vi "Handle Heater PIDs.vi"(7 "DataIndex":i32, 8 "Subtag":string="heater", 10 "HeaterTag":string, 11 "gController in":refnum<class "gController.lvclass">) -> ()   [LabVIEW 2017, in "Controller.lvlib" / "gController.lvclass"]
uses:
  gController.lvclass
  C:/Program Files (x86)/National Instruments/LabVIEW 2017/vi.lib/MSR Consulting, LLC/General Reuse/SuperActor/SuperActor.lvclass
  C:/Program Files (x86)/National Instruments/LabVIEW 2017/vi.lib/ActorFramework/Actor/Actor.lvclass
  <vilib>/Platform/TimedLoop/XDataNode/timing_clust.ctl
  <vilib>/Platform/TimedLoop/XDataNode/nitl_modes.ctl
  <vilib>/Platform/TimedLoop/XDataNode/wakeup.ctl
  <vilib>/MSR Consulting, LLC/General Reuse/SuperActor/SuperActor.lvclass/SuperActor.ctl
  gController.lvclass/gController.ctl
  <vilib>/ActorFramework/Actor/Actor.lvclass/Actor.ctl
  <vilib>/ActorFramework/Message Enqueuer/Message Enqueuer.lvclass/Message Enqueuer.ctl
  Messages/Update Heater DC MSG/Update Heater DC MSG.lvclass
  C:/Program Files (x86)/National Instruments/LabVIEW 2017/vi.lib/ActorFramework/Message/Message.lvclass
  Data/SOAP Data.lvclass
  Data/SOAP Data.lvclass/SOAP Data.ctl
  Data/Read temperatures.vi
  <vilib>/MSR Consulting, LLC/General Reuse/SuperActor/Read CVT Session.vi
  Read DataMap.vi
  Read shutdown.vi
  <vilib>/ActorFramework/Message Enqueuer/Init from Existing Queue.vi
  <vilib>/ActorFramework/Message Priority Queue/Priority Enqueue.vi
  <vilib>/addons/control/pid/pid.llb/PID (DBL).vi
  <vilib>/Platform/TimedLoop/XDataNode/XDataNode.xnode
  <vilib>/ActorFramework/Message Enqueuer/Message Enqueuer.lvclass
  <vilib>/MSR Consulting, LLC/General Reuse/Session APIs/_Session Fwk/Session - Root.lvclass
  <vilib>/Platform/TimedLoop/XDataNode/XDNodeRunTimeDep.lvlib
  <vilib>/ActorFramework/Actor/Actor.lvclass
  <vilib>/MSR Consulting, LLC/General Reuse/Session APIs/CVT/CVT.lvclass
  <vilib>/addons/control/pid/NI_PID_pid.lvlib
  <vilib>/ptbypt/NI_PtbyPt.lvlib
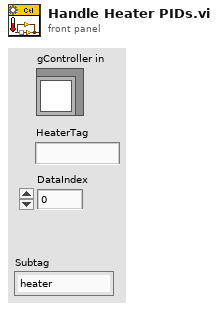
[diagram p1: front panel]
types:
  T1 = typedef "Session - Root.lvclass/Session Handle.ctl" = refnum<data-value>
  T2 = typedef "XDNodeRunTimeDep.lvlib/timing_clust.ctl" = cluster{"Expected End [f-1]":u64, "Actual End [f-1]":u64, "Finished Late? [f-1]":bool, "Expected End [i-1]":u64, "Actual End [i-1]":u64, "Finished Late? [i-1]":bool, "Expected Start [i]":u64, "Actual Start [i]":u64, "Expected Start [f]":u64, "Actual Start [f]":u64, "Source Name":string, "Structure Name":string, "Period":i64, "Deadline":i64, "Offset":i64, "Start":i64, "Priority":i32, "Timeout":i32, "Mode":T3, "Wakeup Reason":T4, "Error":errorcluster, "Source Type":string, "Secondary Source Type":string, "Global End Time":u64, "Global Start Time":u64, "Frame Duration":u64, "Iteration Duration":u64, "Assigned CPU":i32, "I/O Scan Engine Mode":u32}
  T3 = typedef "XDNodeRunTimeDep.lvlib/nitl_modes.ctl" = enum32{"No Change", "Process missed periods, maintain original phase", "Discard missed periods, maintain original phase", "Process missed periods, ignore original phase", "Discard missed periods, ignore original phase"}
  T4 = typedef "XDNodeRunTimeDep.lvlib/wakeup.ctl" = enum32{"Normal", "Aborted", "Asynchronous wakeup", "Timing source error", "Timed loop error", "Timeout"}
  T5 = cluster{"pas_cell_1":sgl, "pas_cell_2":sgl, "pas_las_head_1":sgl, "pas_las_head_2":sgl, "cjc0":sgl, "box_exit":sgl, "crd_heater":sgl, "box_inlet":sgl, "crd_laser_head":sgl, "cjc1":sgl}
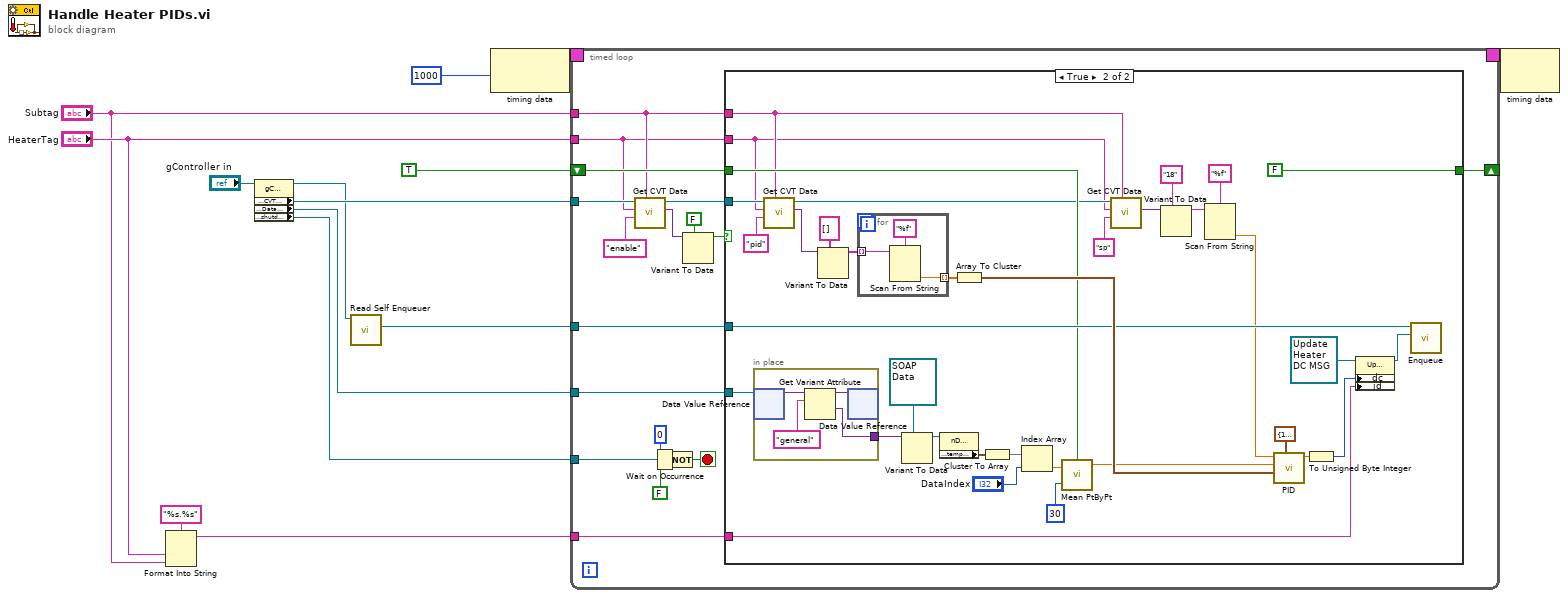
[diagram p0: block diagram]
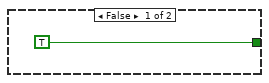
[diagram p2: hidden frame]
diagram:
  n1 = Format Into String(format string="%s.%s", "HeaterTag", "Subtag") -> (resulting string=w6:string)  [unwired: 2 in, 1 out]
  n2 = property class="gController"(reference="gController in") -> (reference out=w3:refnum<class "gController.lvclass">, "Accessors:CVT Session"=w12:T1, "Accessors:DataMap"=w10:refnum<data-value>, "Accessors:shutdown"=w2:refnum<k4>)  [unwired: 1 in, 1 out]
  n3 = call <vilib>:"Read Self Enqueuer.vi"("Actor"=w3) -> ("Self Enqueuer"=w11:refnum<class "Message Enqueuer.lvclass">)  [unwired: 10 in]
  n4 = node-c288(i64 1000 ("Period")) -> (w14:T2)
  n5 = timed-loop {
    timing: w14 -> [_]
    timing-out: [_] -> w13
    tunnel: w12 -> [w17]
    tunnel: "HeaterTag" -> [w15]
    tunnel: w11 -> [w23]
    tunnel: w10 -> [w22]
    tunnel: "Subtag" -> [w16]
    tunnel: w6 -> [w21]
    tunnel: w2 -> [w29]
    shift-right: [w19] -> _
    shift-left: TRUE -> [w20]
    stop <- w28 stop-if-true
    n6 = call <vilib>:"Get CVT Data.vi"("Subgroup"=w16, "Variable"="enable", "Group"=w15, "CVT Session In"=w17) -> ("Data Out"=w26:variant, "CVT Session Out"=w18:T1)  [unwired: 4 in, 2 out]
    n7 = Wait on Occurrence(1:FALSE ("ignore previous (T)"), 2:w29, 3:0 ("ms timeout (-1)")) -> (0:w30:bool)
    n8 = Not(x=w30) -> (.not. x?=w28:bool)
    n9 = Variant To Data(type=FALSE, Variant=w26) -> (data=w27:bool)  [unwired: 1 in, 1 out]
    n10 = case shown="True" w27 {
      tunnel: w23 -> [_ w66]
      tunnel: w22 -> [_ w61]
      tunnel: w21 -> [_ w55]
      tunnel: w20 -> [_ w51]
      tunnel: [TRUE FALSE] -> w19
      tunnel: w18 -> [_ w47]
      tunnel: w16 -> [_ w35]
      tunnel: w15 -> [_ w34]
      frame False {
      }
      frame True {
        n11 = in-place {
          in-place-border: [w72] -> w60
          n12 = in-place-dvr #1(w61) -> (w75:variant)  [unwired: 1 out]
          n13 = Get Variant Attribute(Variant=w75, name="general") -> (duplicate Variant=w74:variant, value=w72:variant)  [unwired: 2 in, 2 out]
          n14 = in-place-dvr #1(w74) -> ()  [unwired: 2 out]
        }
        n15 = call <vilib>:"Get CVT Data.vi"("Subgroup"=w35, "Variable"="pid", "Group"=w34, "CVT Session In"=w47) -> ("Data Out"=w42:variant, "CVT Session Out"=w45:T1)  [unwired: 4 in, 2 out]
        n16 = Variant To Data(type=string[] [], Variant=w42) -> (data=w43:string[])  [unwired: 1 in, 1 out]
        n17 = for {
          tunnel: w43 -> [w71] mode=indexing
          tunnel: [w69] -> w39 mode=indexing
          n18 = Scan From String(format string="%f", input string=w71) -> (output 1=w69:dbl)  [unwired: 3 in, 3 out]
        }
        n19 = Variant To Data(type=refnum<class "SOAP Data.lvclass"> refnum ("Controller.lvlib:nData"), Variant=w60) -> (data=w58:refnum<class "SOAP Data.lvclass">)  [unwired: 1 in, 1 out]
        n20 = property class="nData"(reference=w58) -> ("Accessors:temperatures"=w57:T5)  [unwired: 1 in, 2 out]
        n21 = Array To Cluster(array=w39) -> (cluster=w67:cluster{"[0]":dbl, "[1]":dbl, "[2]":dbl})
        n22 = Cluster To Array(cluster=w57) -> (array=w56:sgl[])
        n23 = Index Array(array=w56, index="DataIndex") -> (element=w53:sgl)
        n24 = call <vilib>:"Mean PtByPt.vi"("x"=w53, "sample length"=30, "initialize"=w51) -> ("mean"=w52:dbl)  [unwired: 1 in, 1 out]
        n25 = call <vilib>:"Get CVT Data.vi"("Subgroup"=w35, "Variable"="sp", "Group"=w34, "CVT Session In"=w45) -> ("Data Out"=w40:variant)  [unwired: 4 in, 3 out]
        n26 = Variant To Data(type="18", Variant=w40) -> (data=w37:string)  [unwired: 1 in, 1 out]
        n27 = Scan From String(format string="%f", input string=w37) -> (output 1=w36:dbl)  [unwired: 3 in, 3 out]
        n28 = call-poly <vilib>:"PID.vi"("output range"=cluster{"output high":dbl, "output low":dbl} {"output high"=100.0, "output low"=0.0}, "PID gains"=w67, "process variable"=w52, "setpoint"=w36) -> ("output"=w64:dbl)  [unwired: 6 in, 1 out]
        n29 = To Unsigned Byte Integer(number=w64) -> (unsigned 8bit integer=w63:u8)
        n30 = property class="Update Heater DC MSG"(reference=refnum<class "Update Heater DC MSG.lvclass"> refnum ("Controller.lvlib:Update Heater DC MSG"), "dc"=w63, "id"=w55) -> (reference out=w62:refnum<class "Update Heater DC MSG.lvclass">)  [unwired: 1 in, 1 out]
        n31 = call <vilib>:"Enqueue.vi"("Message"=w62, "Message Enqueuer in"=w66) -> ()  [unwired: 8 in, 2 out]
      }
    }
  }
  n32 = node-c288(w13) -> ()  [unwired: 1 out]
